vi "Cleanup Session.vi"(8 "error in":errorcluster, 11 "Plugin in":refnum<class "StreamReader.lvclass">) -> (0 "error out":errorcluster, 3 "Plugin out":refnum<class "StreamReader.lvclass">)   [LabVIEW 2024, in "StreamReader.lvlib" / "StreamReader.lvclass"]
uses:
  StreamReader.lvclass
  StreamReader.lvclass/StreamReader.ctl
  StreamReader Strings.vi
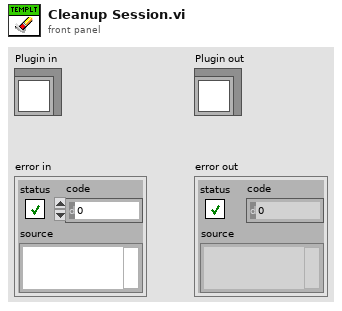
[diagram p1: front panel]
types:
  T1 = typedef "StreamReader.lvlib/StreamReader.lvclass/StreamReader Parameters.ctl" = cluster{"Reader URL":string, "Writer URL":string, "Timeout":i32, "Buffer Size":i32, "Reader endpoint":refnum<k21>, "Channel Names":string[]}
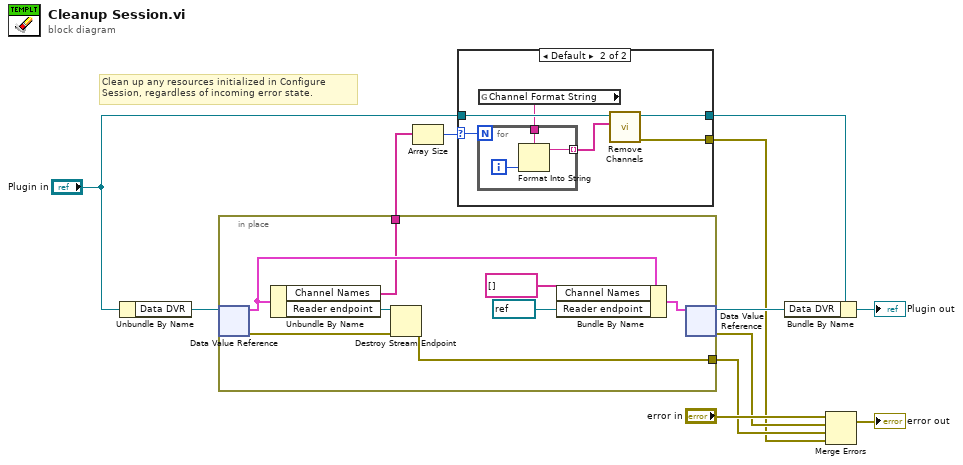
[diagram p0: block diagram]
diagram:
  # "Clean up any resources initialized in Configure Session, regardless of incoming error state."
  n1 = Unbundle By Name("Plugin in") -> ("Data DVR"=w10:refnum<data-value>)
  n2 = in-place {
    in-place-border: [w15] -> w6
    in-place-border: [w13] -> w4
    n3 = in-place-dvr #1(w10) -> (w18:T1, w19:errorcluster)
    n4 = Unbundle By Name(w18) -> ("Channel Names"=w13:string[], "Reader endpoint"=w20:refnum<k21>)
    n5 = Destroy Stream Endpoint(8:w19, 11:w20) -> (0:w15:errorcluster)
    n6 = Bundle By Name(cluster=w18, "Channel Names"=string[] [], "Reader endpoint"=refnum<k21> refnum) -> (w16:T1)
    n7 = in-place-dvr #1(w16) -> (w9:refnum<data-value>, w7:errorcluster)
  }
  n8 = Array Size(array=w4) -> (size(s)=w3:i32)
  n9 = case shown="Default" w3 {
    selector: w3 -> [_ w23]
    tunnel: "Plugin in" -> [w21 w26]
    tunnel: [_ w25] -> w1
    tunnel: [w21 w24] -> w2
    frame 0 {
    }
    frame Default {
      n10 = global read "StreamReader Strings.vi" "Channel Format String"() -> (w22:string)
      n11 = for {
        N: w23 -> [_]
        tunnel: [w30] -> w27 mode=indexing
        tunnel: w22 -> [w28]
        i -> [w29]
        n12 = Format Into String(format string=w28, w29) -> (resulting string=w30:string)  [unwired: 2 in, 1 out]
      }
      n13 = call-dynamic "Remove Channels.vi"("Unique Channel Identifiers to Delete"=w27, "Plugin in"=w26) -> ("error out"=w25:errorcluster, "Plugin out"=w24:refnum<class "StreamReader.lvclass">)  [unwired: 8 in]
    }
  }
  n14 = Bundle By Name(cluster=w2, "Data DVR"=w9) -> (→"Plugin out":refnum<class "StreamReader.lvclass">)
  n15 = Merge Errors("error in", w7, w6, w1) -> (→"error out":errorcluster)
